vi "incrementDataIndex.vi"(8 "error in (no error)":errorcluster, 10 "Count":i32, 11 "FrameParser in":refnum<class "FrameParser.lvclass">) -> (0 "error out":errorcluster, 3 "FrameParser out":refnum<class "FrameParser.lvclass">)   [LabVIEW 2015]
uses:
  FrameParser.lvclass
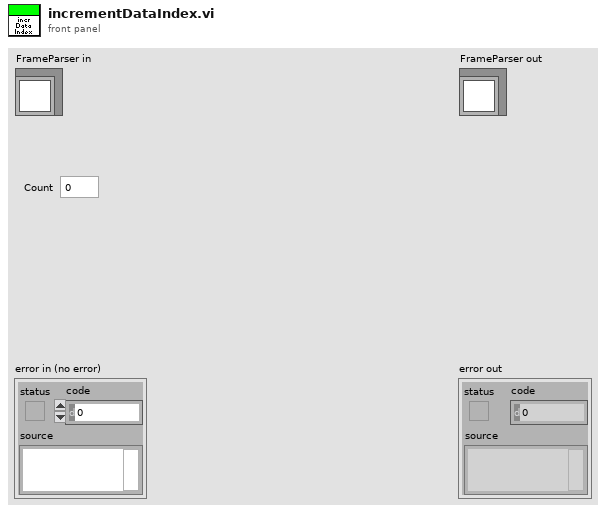
[diagram p1: front panel]
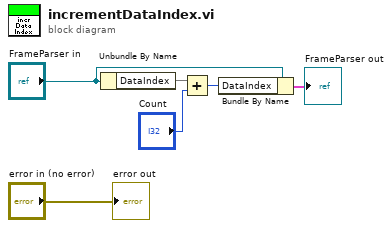
[diagram p0: block diagram]
diagram:
  n1 = Unbundle By Name("FrameParser in") -> ("DataIndex"=w6)
  n2 = Add(x=w6, y="Count") -> (x+y=w4:i32)
  n3 = Bundle By Name(cluster="FrameParser in", "DataIndex"=w4) -> (→"FrameParser out":cluster{})
  "error out" <- "error in (no error)"
